vi "startTest.vi"(8 "error in (no error)":errorcluster, 10 "test":refnum<class>, 11 "TestTestResult in":refnum<class "_TextTestResult.lvclass">) -> (0 "error out":errorcluster, 3 "TestTestResult out":refnum<class "_TextTestResult.lvclass">)   [LabVIEW 2013, in "_TextTestResult.lvclass"]
uses:
  _TextTestResult.lvclass
  TestResult/TestResult.lvclass
  _TextTestResult.lvclass/_TextTestResult.ctl
panel:
  # "JKI VI Tester for LabVIEW\nhttp://jkisoft.com/vi-tester\nCopyright (C) 2007-2009, JKI <info@jkisoft.com>\nALL RIGHTS RESERVED"
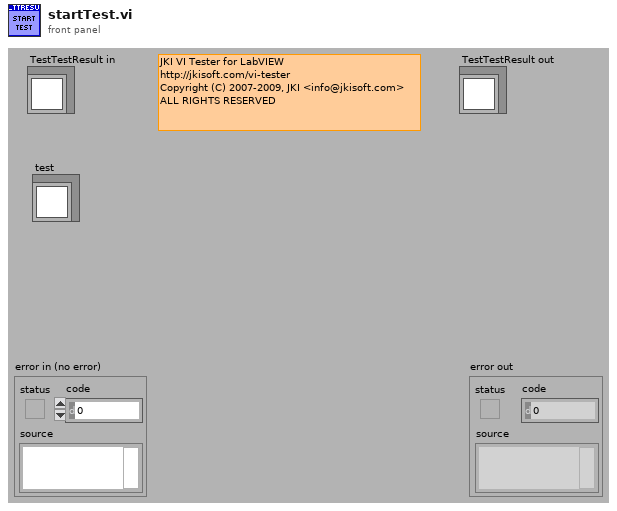
[diagram p1: front panel]
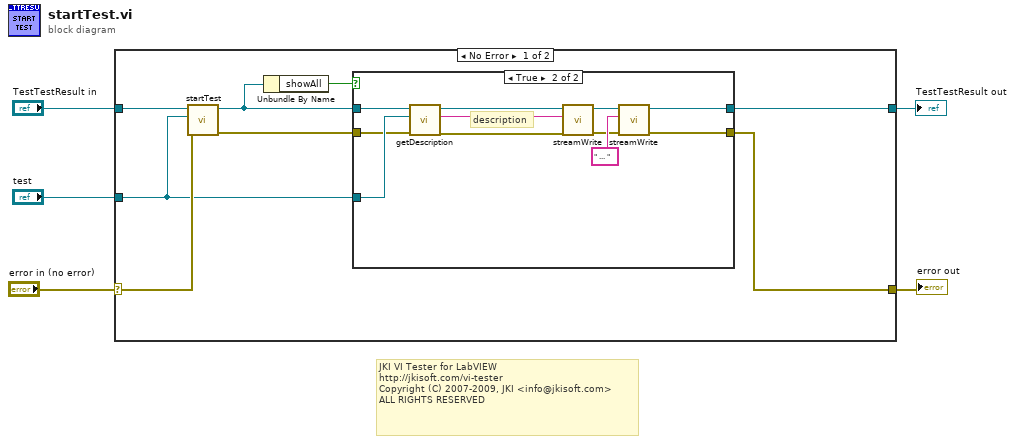
[diagram p0: block diagram]
diagram:
  # "JKI VI Tester for LabVIEW\nhttp://jkisoft.com/vi-tester\nCopyright (C) 2007-2009, JKI <info@jkisoft.com>\nALL RIGHTS RESERVED"
  n1 = case shown="No Error" "error in (no error)" {
    selector: "error in (no error)" -> [w12 w28]
    tunnel: [w7 w28] -> w4
    tunnel: [w9 w27] -> w2
    tunnel: "TestTestResult in" -> [w13 w27]
    tunnel: "test" -> [w11 _]
    frame No Error {
      n2 = call-parent "startTest.vi"("error in (no error)"=w12, "test"=w11, "TestResult in"=w13) -> ("error out"=w8:errorcluster, "TestResult in"=w10:refnum<class "_TextTestResult.lvclass">)  [unwired: 7 in]
      n3 = Unbundle By Name(w10) -> ("showAll"=w6:bool)
      n4 = case shown="True" w6 {
        tunnel: w11 -> [_ w26]
        tunnel: w10 -> [w14 w25]
        tunnel: [w14 w20] -> w9
        tunnel: w8 -> [w15 w24]
        tunnel: [w15 w17] -> w7
        frame False {
        }
        frame True {
          # "description"
          n5 = call-dynamic "getDescription.vi"("error in (no error)"=w24, "test"=w26, "TestTestResult in"=w25) -> ("error out"=w16:errorcluster, "description"=w22:string, "TestTestResult in"=w23:refnum<class "_TextTestResult.lvclass">)  [unwired: 6 in]
          n6 = call "streamWrite.vi"("error in (no error)"=w16, "String"=w22, "TestTestResult in"=w23) -> ("error out"=w18:errorcluster, "TestTestResult out"=w21:refnum<class "_TextTestResult.lvclass">)  [unwired: 7 in]
          n7 = call "streamWrite.vi"("error in (no error)"=w18, "String"=" ... " ("element"), "TestTestResult in"=w21) -> ("error out"=w17:errorcluster, "TestTestResult out"=w20:refnum<class "_TextTestResult.lvclass">)  [unwired: 7 in]
        }
      }
    }
    frame Error {
    }
  }
  "error out" <- w4
  "TestTestResult out" <- w2
